vi "第一次课堂实验《简易示波器》18.vi"() -> ()   [LabVIEW 2018]
uses:
  <vilib>/measure/NI_MABase.lvlib
  <vilib>/measure/NI_MAPro.lvlib
  <vilib>/Waveform/WDTOps.llb/WDT Get XY Value DBL.vi
  <vilib>/measure/mascope.llb/Pulse Measurements 1 chan.vi
  <vilib>/measure/mascope.llb/Amplitude and Levels 1 chan.vi
panel:
  in  "开关":bool
  out "频率":dbl
  out "low state level":dbl caption="低状态电平" format="%.2g"
  out "high state level":dbl caption="高状态电平" format="%.2g"
  out "duty cycle":dbl caption="占空比" format="%.2g"
  out "pulse duration":dbl caption="脉冲持续期" format="%.2g"
  out "period":dbl caption="周期" format="%.2g"
  out "amplitude 2":dbl caption="幅值" format="%.2p"
  out "Y value":dbl caption="Y值" format="%0.2f"
  out "actual Y position":dbl caption="实际Y位置" format="%0.2f"
  out "X value":timestamp caption="X值"
  out "Y":dbl[](array[numeric])
  out "t0":timestamp
  out "dt":dbl
  out "phase out":dbl caption="相位输出" format="%.2p"
  out "error out":errorcluster caption="错误输出"
  in  "frequency":dbl=10.0 caption="频率" format="%0.2p"
  in  "amplitude":dbl=1.0 caption="幅值" format="%0.2p"
  in  "phase":dbl caption="相位" format="%.2p"
  in  "error in (no error)":errorcluster caption="错误输入（无错误）"
  in  "sampling info":cluster{"Fs":dbl, "#s":dbl}={"Fs"=1000.0, "#s"=1000.0} caption="采样信息" {"Fs" format="%.2p"}
  in  "square wave duty cycle (%)":dbl=50.0 caption="方波占空比(%)" format="%0.2f"
  in  "offset":dbl caption="偏移量" format="%0.2p"
  in  "signal type":T1(ring) caption="信号类型"
  out "示波屏":waveform(dbl)(graph)
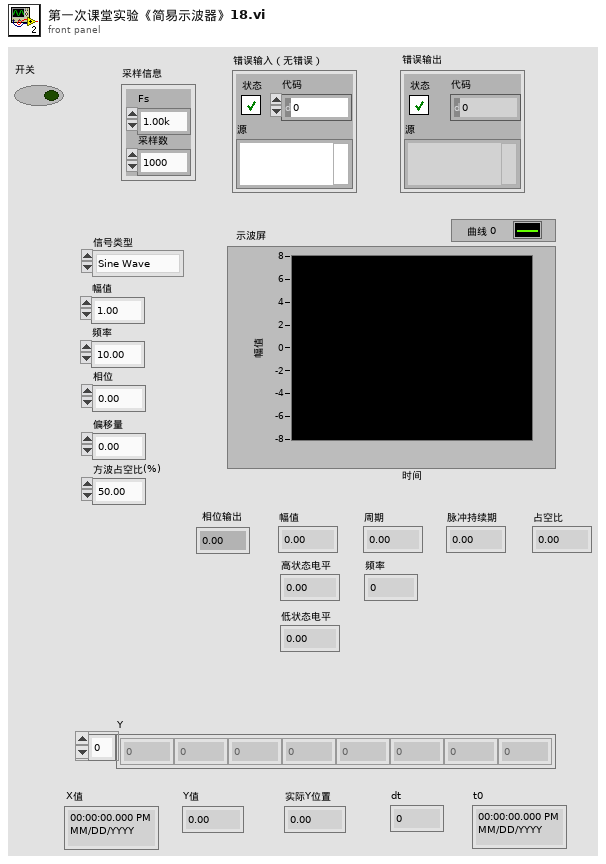
[diagram p1: front panel]
types:
  T1 = enum16{"Sine Wave", "Triangle Wave", "Square Wave", "Sawtooth Wave"}
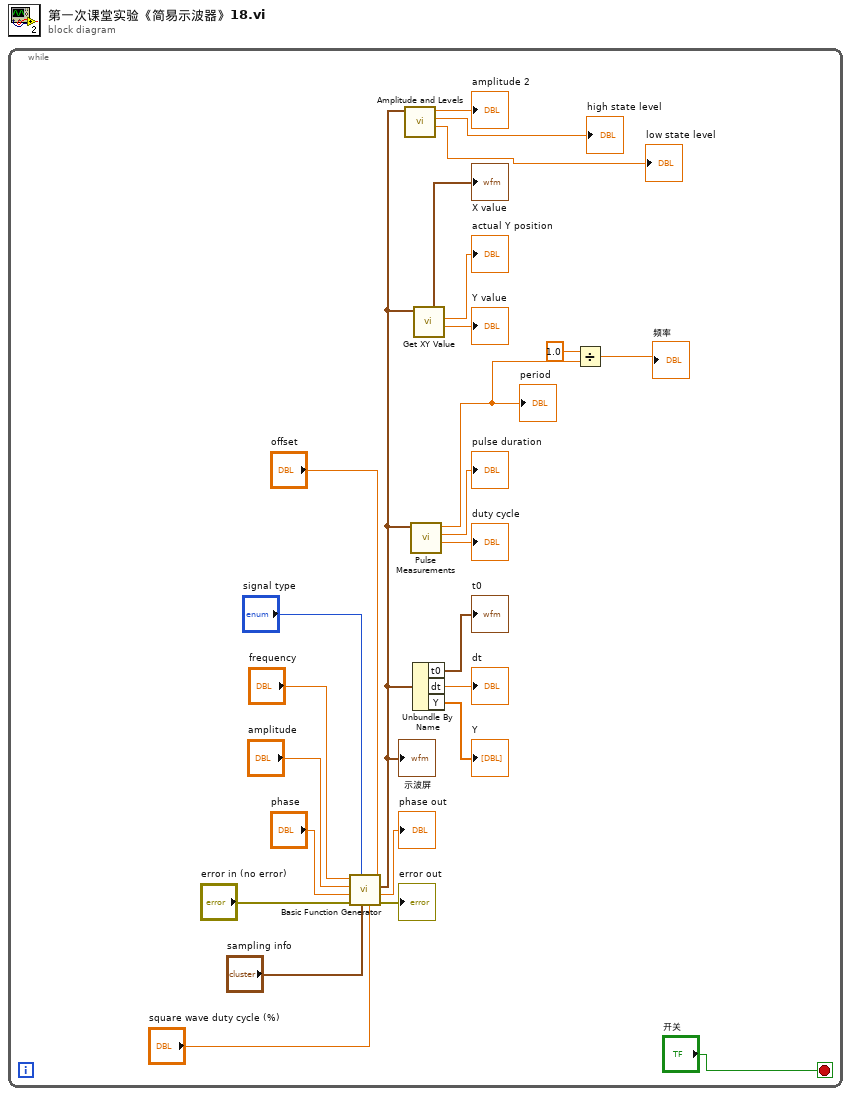
[diagram p0: block diagram]
diagram:
  n1 = while {
    stop <- "开关" stop-if-true
    n2 = call <vilib>:"Basic Function Generator.vi"("offset"="offset", "square wave duty cycle (%)"="square wave duty cycle (%)", "sampling info"="sampling info", "signal type"="signal type", "error in (no error)"="error in (no error)", "phase"="phase", "amplitude"="amplitude", "frequency"="frequency") -> ("error out"=→"error out":errorcluster, "phase out"=→"phase out":dbl, "signal out"=w9:waveform(dbl))  [unwired: 1 in]
    "示波屏" <- w9
    n3 = call-poly <vilib>:"Amplitude and Levels.vi"("signal in"=w9) -> ("low state level"=→"low state level":dbl, "high state level"=→"high state level":dbl, "amplitude"=→"amplitude 2":dbl)  [unwired: 7 in, 1 out]
    n4 = call-poly <vilib>:"Pulse Measurements.vi"("signal in"=w9) -> ("duty cycle"=→"duty cycle":dbl, "pulse duration"=→"pulse duration":dbl, "period"=w4:dbl)  [unwired: 6 in, 2 out]
    "period" <- w4
    n5 = Unbundle By Name(w9) -> ("t0"=→"t0":timestamp, "dt"=→"dt":dbl, "Y"=→"Y":dbl[])
    n6 = call-poly <vilib>:"Get XY Value.vi"("waveform in"=w9) -> ("Y value"=→"Y value":dbl, "actual Y position"=→"actual Y position":dbl, "X value"=→"X value":timestamp)  [unwired: 6 in, 2 out]
    n7 = Divide(x=1.0, y=w4) -> (x/y=→"频率":dbl)
  }
